vi "setSerializedData.vi"(0 "reference":refnum<class "ActorNode.lvclass">, 1 "parent":refnum<class "AbstractNode.lvclass">, 2 "children":refnum<class "AbstractNode.lvclass">[](array[class]), 3 "xmlOut":string, 5 "error in (no error)":errorcluster) -> (14 "reference out":refnum<class "ActorNode.lvclass">, 19 "error out":errorcluster)   [LabVIEW 2016, in "ActorNode.lvclass"]
uses:
  <resource>/Framework/Providers/Open_GDS/UML/ActorNode_class/ActorNode.lvclass
  C:/Program Files (x86)/National Instruments/LabVIEW 2016/resource/Framework/Providers/Open_GDS/UML/RectangularNode_class/RectangularNode.lvclass
  C:/Program Files (x86)/National Instruments/LabVIEW 2016/resource/Framework/Providers/Open_GDS/UML/AbstractNode_class/AbstractNode.lvclass
  <resource>/Framework/Providers/Open_GDS/UML/AbstractNode_class/AbstractNode.lvclass
  <resource>/Framework/Providers/Open_GDS/UML/General/Rectangle/Rectangle Rectangle2D.ctl
  <resource>/Framework/Providers/Open_GDS/UML/MultiLineString_class/MultiLineString.lvclass
  <resource>/Framework/Providers/Open_GDS/UML/RectangularNode_class/RectangularNode.lvclass
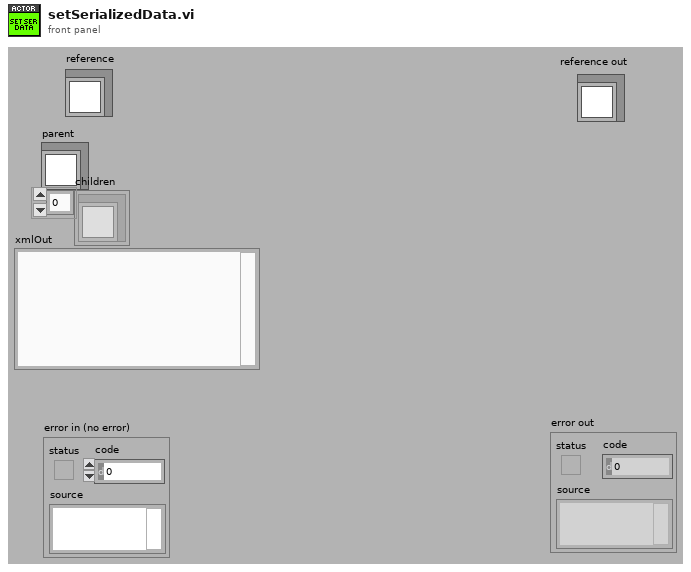
[diagram p1: front panel]
types:
  T1 = typedef "Rectangle Rectangle2D.ctl" = cluster{"x":dbl, "y":dbl, "width":dbl, "height":dbl}
  T2 = cluster{"Base class":cluster{"Base class":cluster{"parent":refnum<k1>, "children":refnum<k1>[]}, "bounds":T1}, "name":refnum<k1>, "DEFAULT_WIDTH":i32, "DEFAULT_HEIGHT":i32, "DEFAULT_GAP":i32}
  T3 = cluster{"Attributes":cluster{"Base class":cluster{"Base class":cluster{"parent":refnum<k1>, "children":refnum<k1>[]}, "bounds":T1}, "name":refnum<k1>, "DEFAULT_WIDTH":i32, "DEFAULT_HEIGHT":i32, "DEFAULT_GAP":i32}, string}
  T4 = typedef "ActorNode.lvclass/ObjectAttributes.ctl" = cluster{"name":refnum<class "MultiLineString.lvclass">, "DEFAULT_WIDTH":i32, "DEFAULT_HEIGHT":i32, "DEFAULT_GAP":i32}
  T5 = typedef "RectangularNode.lvclass/ObjectAttributes.ctl" = cluster{"bounds":T1}
  T6 = typedef "AbstractNode.lvclass/ObjectAttributes.ctl" = cluster{"parent":refnum<class "AbstractNode.lvclass">, "children":refnum<class "AbstractNode.lvclass">[], "Hidden":bool}
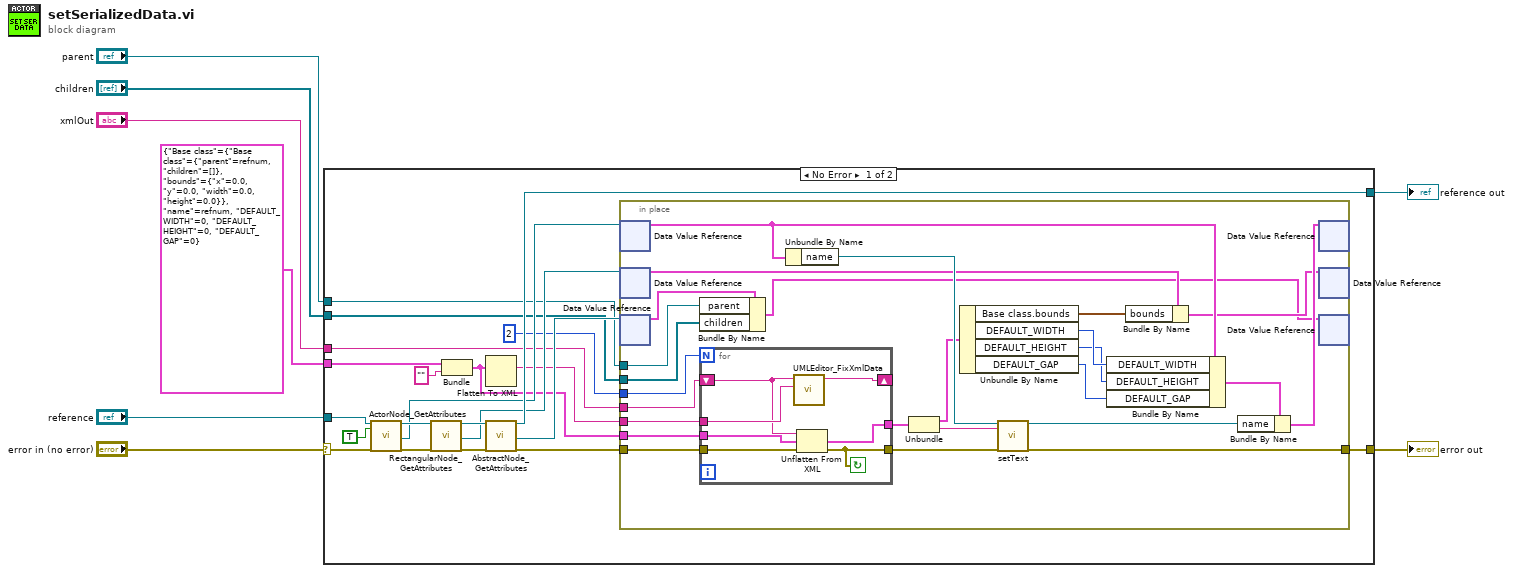
[diagram p0: block diagram]
diagram:
  n1 = case shown="No Error" "error in (no error)" {
    selector: "error in (no error)" -> [w28 w62]
    tunnel: "reference" -> [w29 w63]
    tunnel: [w27 w62] -> w6
    tunnel: [w26 w63] -> w5
    tunnel: "xmlOut" -> [w11 _]
    tunnel: "parent" -> [w10 _]
    tunnel: "children" -> [w9 _]
    tunnel: T2 {"Base class"={"Base class"={"parent"=refnum, "children"=[]}, "bounds"={"x"=0.0, "y"=0.0, "width"=0.0, "height"=0.0}}, "name"=refnum, "DEFAULT_WIDTH"=0, "DEFAULT_HEIGHT"=0, "DEFAULT_GAP"=0} ("Attributes") -> [w24 _]
    frame No Error {
      n2 = call <resource>:"ActorNode_GetAttributes.vi"("reference in"=w29, "OnlyGetDvrReference(False)"=TRUE, "error in (no error)"=w28) -> ("reference out"=w22:refnum<class "ActorNode.lvclass">, "DataRef"=w18:refnum<data-value>, "error out"=w21:errorcluster)  [unwired: 13 in, 1 out]
      n3 = call <resource>:"RectangularNode_GetAttributes.vi"("reference in"=w22, "error in (no error)"=w21) -> ("reference out"=w20:refnum<class "ActorNode.lvclass">, "DataRef"=w17:refnum<data-value>, "error out"=w19:errorcluster)  [unwired: 14 in, 1 out]
      n4 = Bundle("Attributes"=w24, "") -> (w12:T3)  [unwired: 1 out]
      n5 = Flatten To XML(anything=w12) -> (xml string=w13:string)
      n6 = call <resource>:"AbstractNode_GetAttributes.vi"("reference in"=w20, "error in (no error)"=w19) -> ("reference out"=w26:refnum<class "ActorNode.lvclass">, "DataRef"=w16:refnum<data-value>, "error out"=w14:errorcluster)  [unwired: 14 in, 1 out]
      n7 = in-place {
        in-place-border: [w42] -> w27
        in-place-border: 2 -> [w39]
        in-place-border: w14 -> [w38]
        in-place-border: w13 -> [w37]
        in-place-border: w12 -> [w36]
        in-place-border: w11 -> [w35]
        in-place-border: w10 -> [w32]
        in-place-border: w9 -> [w31]
        n8 = in-place-dvr #1(w18) -> (w54:T4)  [unwired: 1 out]
        n9 = in-place-dvr #2(w17) -> (w40:T5)  [unwired: 1 out]
        n10 = in-place-dvr #3(w16) -> (w33:T6)  [unwired: 1 out]
        n11 = Bundle By Name(cluster=w33, "parent"=w32, "children"=w31) -> (w30:T6)
        n12 = for {
          N: w39 -> [_]
          tunnel: w38 -> [w61]
          tunnel: [w57] -> w43
          tunnel: [w60] -> w41
          tunnel: w37 -> [w59]
          tunnel: w36 -> [w58]
          shift-right: [w56] -> _
          shift-left: w35 -> [w55]
          stop <- w57 continue-if-true
          n13 = call <resource>:"UMLEditor_FixXmlData.vi"("XmlTemplateIn"=w59, "xmlIn"=w55) -> ("XML OUt"=w56:string)  [unwired: 9 in]
          n14 = Unflatten From XML(xml string=w55, type=w58, error in (no error)=w61) -> (value=w60:T3, error out=w57:errorcluster)
        }
        n15 = Unbundle By Name(w54) -> ("name"=w49:refnum<class "MultiLineString.lvclass">)
        n16 = Unbundle(w41) -> ("Attributes"=w46:T2, w44:string)
        n17 = Unbundle By Name(w46) -> ("Base class.bounds"=w45:T1, "DEFAULT_WIDTH"=w53:i32, "DEFAULT_HEIGHT"=w52:i32, "DEFAULT_GAP"=w51:i32)
        n18 = call-dynamic "setText.vi"("reference"=w49, "text"=w44, "error in (no error)"=w43) -> ("reference out"=w48:refnum<class "MultiLineString.lvclass">, "error out"=w42:errorcluster)  [unwired: 15 out]
        n19 = Bundle By Name(cluster=w54, "DEFAULT_WIDTH"=w53, "DEFAULT_HEIGHT"=w52, "DEFAULT_GAP"=w51) -> (w50:T4)
        n20 = Bundle By Name(cluster=w40, "bounds"=w45) -> (w34:T5)
        n21 = Bundle By Name(cluster=w50, "name"=w48) -> (w47:T4)
        n22 = in-place-dvr #1(w47) -> ()  [unwired: 2 out]
        n23 = in-place-dvr #2(w34) -> ()  [unwired: 2 out]
        n24 = in-place-dvr #3(w30) -> ()  [unwired: 2 out]
      }
    }
    frame Error {
    }
  }
  "reference out" <- w5
  "error out" <- w6
